vi "collision_fixed_steer2.vi"(6 "safe  dist":dbl=10.0 format="%#_13g", 7 "y":dbl=0.2 format="%#_13g", 8 "obsclose":bool=TRUE, 11 "Max. Vel.":dbl=30.0) -> (0 "collision":bool=TRUE, 1 "collision dist":dbl=nan, 3 "speed limit":dbl)   [LabVIEW 2015]
uses:
  G_ALL.vi
  G_SEN.vi
panel:
  in  "safe time":dbl=0.5
  out "straight":bool
  out "an":dbl=-2.25694
  out "col point":dbl[](array[numeric])=[nan, -21.3]
  out "coldist":dbl=nan
  out "V":dbl=3.694375
  out "Rmax":dbl=-inf
  out "Rmin":dbl=-inf
  out "sensor":dbl[][](array[numeric])=[[-1.5304583967165966, 6.569624655213078, 0.4487461947280802], [-1.5123803553800648, 6.600839252564809, 0.44873888391016814], [-1.5798868335412573, 6.600702497017339, 0.4487279176833], [-1.5216886216577719, 9.603159710523432, 0.44770074776665436], [-1.5313655877780465, 9.6419719017331, 0.4492287086950086], [-1.523389300316294, 12.60341549398873, 0.4466260575335802], [-1.5233893907854144, 12.603416034610877, 0.44887535248893035], [5.990087584334978, 10.963494447794808, 0.45116607548005816], [6.221741073596072, 10.980830526279878, 0.45355671291422156], [5.9936071270446645, 11.240850869489245, 0.45119288181293304], [-1.5383654223459522, 15.592540246828664, 0.4514853145352047], [-9.871601236033586, 12.081252035494268, 0.44840624166361964], [-9.818809426655438, 12.186948767622127, 0.44840258625459123], [-9.44735320706394, 13.283020631001266, 0.4450286438197932], [-9.81432610750644, 13.144511405171443, 0.4483233857256427], [-9.743931372418091, 13.243931372418093, 0.4483209487862904], [-9.847775090309504, 13.52116873622569, 0.44828805010503486], [-9.829415869027697, 13.678658099232255, 0.4482758654082735], [-9.704836591647034, 13.907163096784867, 0.4482661176508645], [-9.822819722231719, 13.851092197505649, 0.4482612437721599], [-9.694719407317505, 14.079929704686844, 0.4482514960147509], [-9.615406741998342, 14.178991062836355, 0.44824905907539864], [-9.607990627804794, 14.359857870824094, 0.4482332189696089], [5.980066449660152, 16.775255255935654, 0.4517740918484479], [-9.552219391192397, 14.488571406471639, 0.4482259081515521], [-9.598842083064628, 14.738800088139001, 0.4481991018186772], [-9.564679561133818, 14.89874122899364, 0.4481869171219159], [-1.4309769895232571, 18.36126424873973, 0.4445424744286406], [-1.50382270432675, 18.434476461172622, 0.4554867688430077], [-9.636584965672458, 15.190112351544258, 0.44815401844066033], [-1.5218566445901764, 18.61357168003814, 0.4518508554380442], [-1.4568554274926686, 18.630022102865794, 0.44814792609227966], [-9.609722299994765, 15.367018743355008, 0.4481393968045468], [-9.56182474777314, 15.520861200018116, 0.4481284305774616], [-9.462716805510386, 15.611725193025839, 0.44812721210778544], [-9.460152536569574, 15.82871081660556, 0.4481064981232912], [-9.472568394095125, 16.0705228348291, 0.44808212872976855], [-9.410096416551857, 16.217015440561624, 0.4480723809723595], [-9.433953229262734, 16.484722663327872, 0.4480443561698085], [-9.366738606084954, 16.63168321360645, 0.44803460841239945], [-9.418125014970215, 16.95047646737776, 0.4479992727917916], [-9.244943886321535, 17.467586586449492, 0.4438771899986423], [-9.42799228252958, 17.477573369517696, 0.4479456601260418], [-9.393967420276597, 17.692736586225667, 0.4479261646112237], [-9.198568680340516, 17.938860587655174, 0.443741939867269], [-9.356898552098706, 17.908360250344202, 0.4479066690964056], [-9.31677513957232, 18.124407561833465, 0.44788717358158747], [-9.358374136887987, 18.476529266946585, 0.44784818255195125], [-9.290024411686542, 18.659942009678325, 0.4478335609158377], [-1.4789544873589022, 21.298658685480213, 0.45652856039547757], [-9.322189086670184, 19.014728027537103, 0.4477945698862015], [-1.4295247135494842, 21.663833685781242, 0.4477799482500879], [-1.5104216938102306, 21.677354630622453, 0.4522224886892644], [-9.308253507600966, 19.302278685191865, 0.4477653266139743], [-9.309999930888686, 19.625392898761945, 0.4477312094630426], [-9.267411332352088, 19.880094075993874, 0.44770684006952], [-9.259863677965905, 20.20523628235378, 0.4476727229185883], [-10.761395333704177, 19.60556627074318, 0.4523601757626673], [-10.65333737048856, 19.74903988749979, 0.45236748658072407], [-9.28550940572247, 20.601780885449482, 0.44762885801024754], [-9.229810855854572, 20.858749546746573, 0.4476044886167249], [-10.560231191577744, 20.2369534672775, 0.45241135148906486], [-10.59794834367646, 20.626093684277787, 0.45245399792772945], [-10.46884427196551, 20.752121422111667, 0.45245887180643396], [-1.481627491326594, 24.688260270230966, 0.4474119704078961], [2.41453226692714, 27.47874111184458, 0.45293651191947765], [2.2051889934181257, 27.49889857639732, 0.45293651191947765], [-1.3984167404305334, 30.183380970562354, 0.44674424902537585], [-9.27247533961122, 28.63414421014917, 0.4597928405932163], [-1.4542170646867847, 33.77509436961648, 0.4536931815883555], [-12.254333639737276, 34.21572986135418, 0.46208843741760597], [9.646867745895442, 40.14137035344789, 0.4546167816028634], [9.346440466929042, 40.30169736837388, 0.4546265293602724], [9.995186075205359, 40.161918033340946, 0.45463018476930084], [9.687603481990763, 40.29609551732546, 0.4639088310777111], [10.355453085480514, 40.217666998138846, 0.4546484618144428], [9.398132099956998, 40.50523366028126, 0.46395635139413954], [9.081977878364448, 40.614980212047534, 0.4546557726324996], [10.748232349142603, 40.37551463322397, 0.45468014202602225], [9.129514514304716, 40.80924640889365, 0.46404042580012833], [-19.28793420922692, 37.246885664560835, 0.4642085746121059], [9.064874855356468, 41.997147100113274, 0.4644571424211163], [-18.15469952147041, 38.74952730488572, 0.4644936965106766], [-17.918417740569364, 39.049489362133144, 0.46455218305397317], [-17.647317560719458, 39.28521999634086, 0.46458508173457747], [-17.399531396582823, 39.572962074832176, 0.464639912868918], [-17.17365632105936, 39.91336172321326, 0.4647166764569947], [-22.342947610202373, 37.578658573998304, 0.4648957914958404], [-22.10962516766409, 37.87326216337433, 0.4649396564033128], [-21.83550453243502, 38.10718015201812, 0.464957933448093], [-21.55372087277477, 38.330424808794795, 0.4649725550839171], [-21.274889895785886, 38.55993347394059, 0.4649908321286973], [-21.029483225367702, 38.84738334349325, 0.46503469703616973], [-20.78067516476939, 39.13321220902357, 0.4650785619436421], [-20.26312153109795, 39.6824069959594, 0.46515898094067487], [-17.797224253682096, 42.105163740090134, 0.46553914347210246], [-17.23352970768187, 42.66617557482583, 0.46564149492287144], [-16.938457745789194, 42.925328193479906, 0.46568535983034387], [17.322133973531134, 42.86754408677865, 0.4657219139199042], [-16.655640004933225, 43.219193196203896, 0.4657438463736404], [-14.15297871173657, 45.19333081613475, 0.4660947656334197], [-14.06731724741144, 46.160481898838114, 0.4664200970305068], [-13.150394836379569, 47.19397827432551, 0.4666796310663852], [-12.785386796883316, 47.364674916290646, 0.46670156352012143], [-12.459115816412385, 47.67669240177406, 0.46677832710819817], [-12.136259424266495, 48.015284147391746, 0.466866056923143], [-9.972349925099477, 49.42985893516836, 0.4671804220933619], [-10.436781004884613, 49.62393525530377, 0.4672864289530869], [-8.077970793908602, 50.511020876260254, 0.46743630072028436], [-10.017137069339602, 51.65924357399377, 0.4679809566547335], [-9.703791968771103, 52.28425658797661, 0.46818200414731537], [-7.575744126121782, 52.72039993287564, 0.4682039366010516], [5.9133064222073175, 53.46127369852273, 0.45613012094061905], [6.356642028184218, 53.46728894444298, 0.4561374317586759], [8.099817339627355, 53.2347435881879, 0.4684196057294576], [8.536907918677832, 53.18187761786749, 0.4684269165473697], [8.977251802514107, 53.14485282772466, 0.4561471795160849], [5.492333795510142, 53.65014189103438, 0.4561471795160849], [9.00928110542982, 53.321977193221436, 0.46850733554440244], [6.832896586246616, 53.7071746478883, 0.4561739858489598], [1.989687447899467, 54.14092718075492, 0.45617520431863595], [-4.637301999436954, 53.96739335484715, 0.45617520431863595], [7.7156976320662, 53.629692461756065, 0.46854023422500674], [10.861374957060782, 53.52445996847586, 0.45623734627211865], [10.444784718162802, 53.715238928850184, 0.4687485925355007], [10.89956629047575, 53.70035858509785, 0.468777835807149], [10.086168974376077, 54.20659560913531, 0.4688984643026981], [15.473538348436962, 53.33293737243348, 0.4690739239325878], [15.075545778895796, 53.5905545371459, 0.46912144424901625], [15.965742273424409, 53.3769646950345, 0.4691433767027524], [16.481810034088696, 53.48266167265918, 0.46923841733560934], [-3.937384054853013, 56.48390194101806, 0.45647372938928826], [14.881305971946919, 54.55544784522514, 0.4694394648281912], [17.54943187485922, 53.75385519804383, 0.4694577418729714], [7.748601530003164, 56.941174491550086, 0.4565797362511117], [20.102739641842973, 53.88791487688127, 0.46983059358648693], [20.59848340778603, 53.84940005470817, 0.46988542472082745], [19.763744907192873, 54.32238571654336, 0.4699329450372559], [21.226563266096697, 54.119607953091055, 0.4700645397596731], [5.15520085107671, 59.60364587126739, 0.47059457405829813], [17.179103122702053, 57.16750291150652, 0.45686607662500267], [5.648602536305274, 59.5963213111867, 0.47060919569412224], [8.262304622246873, 60.484123045962804, 0.47104784476884637], [12.720999304748343, 59.71872759813299, 0.4710697772225826], [7.78089815695139, 60.67295845949319, 0.4710917096763188], [-7.8793393294743455, 61.39629051625974, 0.47135855453010933], [-0.29190538898263213, 70.3993626636003, 0.4581515621333217], [-0.29194900473725677, 70.40935859480476, 0.47445834132482656], [0.8783118563172027, 70.59425088215231, 0.4581759315268444], [0.8790971798389399, 70.65424175329007, 0.4745497265487274], [2.0967743014213513, 72.12797583739979, 0.45836601279632094], [-8.110079882755713, 72.0217189519484, 0.47522232179663776], [5.235520456007894, 83.378606212284, 0.45975384975743505], [-3.240112570543469, 85.96637174877078, 0.4600560302371157], [4.792807940400054, 87.90402618987854, 0.4809028273143153], [4.793942080772132, 87.92399903562121, 0.46030337958137046], [-8.146388565341844, 92.15650677882385, 0.48254410593557473], [-2.802519336461366, 95.22719695016279, 0.4611818962178615], [-3.520704269592428, 164.8515923526585, 0.46966488210309104], [-11.526176157591637, 13.878215627584847, 0.4481101535323196], [-11.789979240029444, 14.885450607304874, 0.44800292820082], [-12.091348233927823, 14.57967932264858, 0.4480017097311439], [-12.030768302326846, 14.71887293974657, 0.4479956173827632], [-11.96142328919889, 14.850966868927898, 0.4479907435040587], [-9.215291856779873, 17.690305061581164, 0.4438150480463897], [-9.236492158493983, 18.281477328454823, 0.44362862218963195], [-9.154174242232312, 18.438254681457707, 0.44359572350902765], [-9.141925218880708, 18.714718570965932, 0.44351164910303886], [-1.414617401462343, 21.474418326335975, 0.4434092976522699], [-9.206745289003786, 19.129951926170946, 0.44336908815375353], [-9.224999383677053, 19.47816763232024, 0.4432557704761165], [-9.183698782366013, 19.732132644809052, 0.44318266229699577], [-9.177445498117294, 20.05654995000434, 0.4430803108462268], [-9.166219172191244, 20.382075606343538, 0.4429779593954578], [-9.070189987043294, 20.558546354351627, 0.44293774989694146], [-9.027184785637978, 20.84106063007659, 0.44285367549095267], [-9.265946030899864, 21.685443023687828, 0.447513103391015], [-9.298762356180521, 22.15043195733767, 0.44746070919494135], [-1.4639438802396605, 27.435270867039012, 0.4412343293234294], [2.307965703554175, 27.469140278750547, 0.44706592501987463], [-9.175563115010997, 28.371452130675763, 0.4532301631114254], [-9.03589297233244, 28.66704646113176, 0.45325818791397643], [-1.4146408027345068, 30.492954521014685, 0.4401194295918389], [-12.23951207009181, 34.17857930362207, 0.45402460534026334], [-12.1194280298934, 38.2047121320138, 0.4544790945294605], [-19.197928435902572, 37.780367863415314, 0.45478736735752184], [-17.90491585155485, 39.02270210519787, 0.4548470723716523], [10.80061477854137, 41.796091299925706, 0.4645448722360611], [-17.64731860873607, 39.285222121508326, 0.4548616940077659], [-17.40387688242602, 39.58197119941406, 0.454881189522584], [-17.173657340946782, 39.91336388568401, 0.4549055589161066], [-22.050119289273855, 37.780749913950906, 0.4549664823999132], [-21.039710335885733, 38.86457357076146, 0.4550140027172824], [-20.498703614653966, 39.36529276030614, 0.4550334982321005], [-19.95622387432352, 39.87539282427752, 0.45505543068627086], [-19.96584246392425, 39.892925198004406, 0.46517360257649903], [-19.71849601752628, 40.19790570184635, 0.46522843371083955], [-17.52126508189382, 42.39576618036936, 0.465593974606443], [-17.2254757973876, 42.64787167133072, 0.4552113948048157], [-16.934511313174397, 42.91614262278823, 0.4552272349106054], [-16.63630544611904, 43.17308550675596, 0.455241856546719], [17.35435473718568, 42.94077134247465, 0.45525038583445193], [-16.368979606633143, 43.51111569166321, 0.4552674444099178], [-16.376551606374004, 43.529624124377364, 0.465809643734849], [-15.482517326111966, 44.36540593305769, 0.46597413713787056], [-14.140121973719118, 45.155456087267005, 0.4553600481053038], [-14.61518532805766, 45.3514634779125, 0.46620442790210076], [-13.967105665492628, 45.85658071417634, 0.4554343747555478], [-12.732220043894518, 47.18226805029135, 0.4555440370263997], [-12.391256444356108, 47.43608121795645, 0.4555623140715417], [-12.081023590373213, 47.8126814545092, 0.45559643122247334], [-11.78806941435407, 48.27422398034609, 0.4669245434664395], [-10.742622242787393, 49.122285505371394, 0.45571096737202976], [-10.786169676183954, 49.30722484276436, 0.46720235454709813], [-10.414711881352668, 49.52640376312698, 0.45574995840166593], [-7.749398570022519, 51.08309165283863, 0.4676227265770421], [-8.230385825965628, 51.39802411465917, 0.45592176262600054], [-10.013064829232125, 51.63966552470979, 0.45599121539754006], [10.051053315658523, 54.03005727127254, 0.45627755577143103], [-9.684327877683424, 54.50882427125252, 0.4563262945584763], [-3.4696359799027956, 56.436415484842804, 0.4564639816318792], [-3.0200247710824435, 56.68432389578455, 0.45649078796475406], [8.73796580135908, 57.15312208792874, 0.45662360115945244], [9.221080416128158, 57.16352701734963, 0.4566345673865376], [11.175859219610716, 57.23001513109769, 0.4566869615826113], [1.9728684167848833, 59.995559676916635, 0.42933597317153727], [-7.872597250938968, 61.34675066002998, 0.4571134259692574], [-8.106554242489338, 71.99193096774223, 0.458403785356281], [3.679295078452094, 87.76971186036354, 0.41916662545584943], [6.462482767471447, 102.0984336178372, 0.48611909589457647], [-4.972546548304975, 22.727410853324365, 0.4427403578133156], [-12.82222968885361, 27.363329920838236, 0.45330083435264107], [-15.118256938908255, 29.423703318743403, 0.4536566274980715], [-18.159279338735963, 38.75841956958901, 0.45483245073553874], [-17.805598505289773, 42.12332889606653, 0.45518215153258856], [-17.541802064902818, 42.441356592102444, 0.45520408398675893], [-15.4754324248608, 44.346705655865925, 0.4553222755453437], [-11.7396957446091, 48.09048791231148, 0.4556183636766437], [-11.088046794705612, 48.813107220413954, 0.4556841610391548], [-9.959619857089923, 49.37122779684034, 0.45571949665976264], [-7.9246084254415505, 52.158920510207636, 0.45600705550332976], [38.47373334497915, 62.182195635275114, 0.47565000464449375], [2.2272997454946832, 105.5757022071159, 0.46244057539330563], [-24.75, -14.799999999999999, 1.31], [-24.75, 28.2, 1.1500000000000001], [-24.5, -14.799999999999999, 1.31], [-24.5, 26.45, 0.36], [-24.5, 26.7, 0.36], [-24.5, 26.95, 0.34], [-24.5, 28.45, 0.29], [-24.5, 28.7, 0.29], [-24.25, -14.799999999999999, 1.32], [-24.0, -14.799999999999999, 1.32], [-24.0, -7.549999999999999, 1.4000000000000001], [-24.0, -1.0499999999999994, 1.44], [-24.0, 6.200000000000001, 1.43], [-23.75, -14.799999999999999, 1.33], [-23.75, -8.049999999999999, 1.4000000000000001], [-23.75, -7.799999999999999, 0.81], [-23.75, -7.549999999999999, 1.41], [-23.75, -1.0499999999999994, 1.44], [-23.75, -0.7999999999999994, 1.44], [-23.75, -0.5499999999999994, 1.44], [-23.75, -0.2999999999999994, 1.44], [-23.75, 5.950000000000001, 0.3], [-23.5, -14.799999999999999, 1.33], [-23.5, -8.049999999999999, 1.41], [-23.5, -7.799999999999999, 1.41], [-23.5, -0.7999999999999994, 1.45], [-23.5, -0.5499999999999994, 1.45], [-23.5, 6.200000000000001, 1.44], [-23.5, 27.7, 0.36], [-23.25, -14.799999999999999, 1.34], [-23.25, 27.7, 1.18], [-23.25, 36.7, 1.02], [-23.0, -14.799999999999999, 1.34], [-23.0, 6.200000000000001, 1.45], [-23.0, 7.450000000000001, 0.34], [-23.0, 27.7, 0.37], [-22.75, -17.55, 1.31], [-22.75, -17.3, 1.31], [-22.75, -17.05, 1.32], [-22.75, -16.8, 1.32], [-22.75, -16.55, 1.32], [-22.75, -16.3, 1.33], [-22.75, -16.05, 1.33], [-22.75, -15.799999999999999, 1.33], [-22.75, -15.549999999999999, 1.34], [-22.75, -15.299999999999999, 1.34], [-22.75, -15.049999999999999, 1.34], [-22.75, -14.799999999999999, 1.35], [-22.75, 6.200000000000001, 1.46], [-22.75, 6.450000000000001, 1.45], [-22.75, 6.700000000000001, 1.45], [-22.75, 6.950000000000001, 1.45], [-22.75, 7.200000000000001, 1.45], [-22.75, 7.450000000000001, 1.45], [-22.75, 7.700000000000001, 1.45], [-22.75, 7.950000000000001, 1.45], [-22.75, 8.200000000000001, 1.44], [-22.75, 8.450000000000001, 1.44], [-22.75, 8.700000000000001, 1.44], [-22.5, 7.700000000000001, 0.37], [-22.5, 7.950000000000001, 0.37], [-20.25, 4.700000000000001, 0.56], [-20.25, 4.950000000000001, 0.56], [-20.0, 8.200000000000001, 1.5], [-20.0, 8.450000000000001, 1.51], [-19.75, 8.450000000000001, 1.51], [-19.0, -9.549999999999999, 0.45], [-18.25, -10.549999999999999, 0.47000000000000003], [-18.25, -10.299999999999999, 0.99], [-18.0, 1.7000000000000006, 0.32], [-18.0, 2.2000000000000006, 0.74], [-18.0, 2.4500000000000006, 0.32], [-17.75, 1.4500000000000006, 0.75], [-17.75, 1.9500000000000006, 0.75], [-17.75, 4.700000000000001, 0.31], [-17.75, 4.950000000000001, 0.31], [-17.5, -5.049999999999999, 0.26], [-17.5, 1.4500000000000006, 0.76], [-17.25, -10.549999999999999, 0.53], [-17.25, -7.049999999999999, 0.65], [-17.25, -6.799999999999999, 0.65], [-17.25, -4.799999999999999, 0.29], [-17.25, -0.2999999999999994, 0.78], [-17.25, -0.04999999999999938, 0.38], [-17.25, 1.4500000000000006, 0.39], [-16.75, -6.299999999999999, 0.28], [-16.75, -5.299999999999999, 0.32], [-16.25, -12.299999999999999, 0.51], [-16.25, -5.799999999999999, 0.76], [-16.25, -0.04999999999999938, 0.48], [-16.25, 4.700000000000001, 0.46], [-16.25, 4.950000000000001, 0.45], [-16.25, 5.200000000000001, 0.45], [-16.0, -5.549999999999999, 0.36], [-16.0, -0.04999999999999938, 0.49], [-16.0, 5.700000000000001, 0.85], [-15.5, -9.799999999999999, 0.22], [-15.5, -9.549999999999999, 0.24], [-15.5, -5.799999999999999, 0.8], [-15.5, -5.299999999999999, 0.42], [-15.5, -5.049999999999999, 0.44], [-15.5, -0.2999999999999994, 0.54], [-15.5, 0.4500000000000006, 0.55], [-15.5, 9.450000000000001, 1.59], [-15.25, -10.049999999999999, 0.66], [-15.25, -9.799999999999999, 0.67], [-15.25, 1.4500000000000006, 0.23], [-15.25, 9.200000000000001, 1.2], [-15.25, 9.950000000000001, 1.59], [-15.0, -21.3, 1.36], [-15.0, 8.950000000000001, 1.61], [-14.75, -19.3, 0.21], [-14.75, -18.8, 0.8300000000000001], [-14.75, -11.799999999999999, 0.62], [-14.75, 4.700000000000001, 0.24], [-14.75, 9.450000000000001, 1.61], [-14.5, -17.8, 0.87], [-14.5, -17.55, 0.33], [-14.5, -17.3, 0.89], [-14.5, -10.299999999999999, 0.68], [-14.5, -10.049999999999999, 0.7000000000000001], [-14.5, -9.799999999999999, 0.71], [-14.5, 8.950000000000001, 0.86], [-14.5, 9.200000000000001, 1.61], [-14.25, -19.05, 0.25], [-14.25, -17.8, 0.33], [-14.25, -17.55, 0.33], [-14.25, -15.049999999999999, 0.46], [-14.25, -6.049999999999999, 0.5], [-14.25, -5.799999999999999, 0.89], [-14.25, -5.299999999999999, 0.53], [-14.25, 0.4500000000000006, 0.34], [-14.25, 8.950000000000001, 1.24], [-14.25, 9.200000000000001, 0.87], [-14.0, -11.049999999999999, 0.26], [-14.0, -10.799999999999999, 0.27], [-14.0, -9.799999999999999, 0.33], [-14.0, -9.549999999999999, 0.35000000000000003], [-14.0, -0.7999999999999994, 0.35000000000000003], [-14.0, -0.2999999999999994, 0.6900000000000001], [-14.0, -0.04999999999999938, 0.36], [-14.0, 0.20000000000000062, 0.6900000000000001], [-14.0, 0.4500000000000006, 0.6900000000000001], [-14.0, 9.200000000000001, 0.87], [-14.0, 9.450000000000001, 1.24], [-13.75, -10.549999999999999, 0.72], [-13.75, -10.299999999999999, 0.31], [-13.75, -10.049999999999999, 0.32], [-13.75, 9.450000000000001, 1.26], [-13.5, -19.05, 0.27], [-13.5, 9.200000000000001, 0.9], [-13.5, 9.450000000000001, 1.26], [-13.5, 19.45, 0.42], [-13.25, -18.8, 0.86], [-13.25, 8.950000000000001, 0.22], [-13.25, 9.200000000000001, 1.28], [-13.25, 9.450000000000001, 1.28], [-13.25, 9.700000000000001, 1.27], [-13.25, 9.950000000000001, 1.27], [-13.25, 14.450000000000001, 1.56], [-13.25, 19.7, 1.47], [-13.25, 27.7, 1.31], [-13.0, -19.8, 0.26], [-13.0, -19.55, 0.27], [-13.0, -19.3, 0.85], [-13.0, 9.450000000000001, 1.28], [-13.0, 9.950000000000001, 1.27], [-13.0, 14.200000000000001, 1.57], [-13.0, 19.7, 1.47], [-12.75, 8.700000000000001, 0.28], [-12.75, 14.450000000000001, 1.58], [-12.75, 19.7, 0.43], [-12.5, 30.7, 1.26], [-12.0, 11.450000000000001, 1.6300000000000001], [-11.75, 10.700000000000001, 1.3], [-11.5, 4.950000000000001, 0.59], [-11.5, 5.200000000000001, 0.58], [-11.5, 5.450000000000001, 0.85], [-11.5, 5.700000000000001, 0.85], [-11.5, 5.950000000000001, 0.27], [-11.5, 10.450000000000001, 0.97], [-11.5, 10.700000000000001, 1.3], [-11.5, 10.950000000000001, 1.31], [-11.5, 11.200000000000001, 1.29], [-11.5, 11.450000000000001, 1.29], [-11.25, 5.200000000000001, 0.32], [-11.25, 6.200000000000001, 0.28], [-11.25, 10.200000000000001, 0.67], [-11.25, 10.450000000000001, 1.32], [-11.25, 10.700000000000001, 1.31], [-11.25, 10.950000000000001, 1.3], [-11.25, 11.200000000000001, 1.3], [-11.0, 3.9500000000000006, 0.68], [-11.0, 10.450000000000001, 0.65], [-11.0, 10.700000000000001, 0.99], [-11.0, 10.950000000000001, 0.98], [-10.75, 3.7000000000000006, 0.45], [-10.75, 3.9500000000000006, 0.7000000000000001], [-10.75, 4.200000000000001, 0.6900000000000001], [-10.75, 4.450000000000001, 0.7000000000000001], [-10.75, 4.700000000000001, 0.6900000000000001], [-10.75, 4.950000000000001, 0.9500000000000001], [-10.75, 5.200000000000001, 0.9500000000000001], [-10.75, 10.700000000000001, 0.67], [-10.75, 10.950000000000001, 1.0], [-10.75, 11.200000000000001, 0.98], [-10.5, 3.9500000000000006, 0.72], [-10.5, 4.200000000000001, 0.48], [-10.5, 4.450000000000001, 0.47000000000000003], [-10.5, 5.200000000000001, 0.7000000000000001], [-10.5, 5.450000000000001, 0.42], [-10.5, 10.450000000000001, 0.72], [-10.5, 10.950000000000001, 0.68], [-10.5, 11.200000000000001, 1.0], [-10.5, 11.450000000000001, 0.99], [-10.5, 11.700000000000001, 0.98], [-10.25, 4.700000000000001, 0.99], [-10.25, 11.200000000000001, 1.01], [-10.25, 11.450000000000001, 0.33], [-10.25, 11.700000000000001, 0.99], [-10.25, 12.200000000000001, 0.96], [-10.25, 15.700000000000001, 0.36], [-10.0, 11.450000000000001, 0.33], [-10.0, 11.700000000000001, 0.99], [-10.0, 11.950000000000001, 1.6600000000000001], [-10.0, 12.200000000000001, 1.6600000000000001], [-10.0, 15.450000000000001, 1.6], [-10.0, 15.700000000000001, 1.59], [-9.75, 11.950000000000001, 1.6600000000000001], [-9.75, 12.200000000000001, 1.6600000000000001], [-9.75, 12.450000000000001, 1.6600000000000001], [-9.75, 12.700000000000001, 0.27], [-9.75, 15.700000000000001, 1.6], [-9.5, 11.950000000000001, 0.66], [-9.5, 12.200000000000001, 0.67], [-9.5, 12.700000000000001, 0.27], [-9.5, 15.950000000000001, 0.38], [-9.5, 16.2, 0.36], [-8.5, -10.549999999999999, 1.31], [-8.5, -1.0499999999999994, 1.79], [-8.5, -0.5499999999999994, 1.79], [-8.5, 6.450000000000001, 0.38], [-8.25, -14.049999999999999, 1.59], [-8.25, -10.549999999999999, 1.32], [-8.25, -1.5499999999999994, 1.59], [-8.25, -1.2999999999999994, 1.59], [-8.25, -1.0499999999999994, 1.8], [-8.25, -0.7999999999999994, 1.8], [-8.25, 2.4500000000000006, 1.8], [-8.25, 6.700000000000001, 1.31], [-8.0, -14.049999999999999, 1.59], [-8.0, -13.799999999999999, 1.6], [-8.0, -10.549999999999999, 1.6600000000000001], [-8.0, -10.299999999999999, 1.6600000000000001], [-8.0, -3.0499999999999994, 1.57], [-8.0, -2.7999999999999994, 1.79], [-8.0, -1.2999999999999994, 1.8], [-8.0, -1.0499999999999994, 1.6], [-8.0, -0.7999999999999994, 1.8], [-8.0, 2.4500000000000006, 1.81], [-8.0, 2.7000000000000006, 1.81], [-8.0, 2.9500000000000006, 1.81], [-8.0, 6.700000000000001, 1.78], [-8.0, 8.950000000000001, 0.46], [-8.0, 9.200000000000001, 0.43], [-8.0, 30.2, 1.3], [-7.75, -14.049999999999999, 0.38], [-7.75, -10.799999999999999, 0.32], [-7.75, -10.549999999999999, 0.66], [-7.75, -3.0499999999999994, 1.79], [-7.75, -2.7999999999999994, 1.79], [-7.75, -1.5499999999999994, 0.24], [-7.75, -1.2999999999999994, 1.8], [-7.75, -1.0499999999999994, 0.25], [-7.75, 2.7000000000000006, 1.81], [-7.75, 6.700000000000001, 1.78], [-7.75, 6.950000000000001, 0.21], [-7.75, 9.200000000000001, 0.2], [-7.5, -16.05, 1.55], [-7.5, -10.799999999999999, 1.6600000000000001], [-7.5, -10.549999999999999, 1.67], [-7.5, -2.5499999999999994, 0.2], [-7.5, 2.7000000000000006, 0.21], [-7.5, 2.9500000000000006, 0.21], [-7.5, 6.700000000000001, 1.78], [-7.5, 6.950000000000001, 1.78], [-7.5, 7.200000000000001, 1.78], [-7.5, 7.450000000000001, 0.42], [-6.75, -13.549999999999999, 0.85], [-6.75, -13.299999999999999, 1.62], [-6.5, -13.549999999999999, 0.48], [-6.5, -13.299999999999999, 1.62], [-6.25, -13.299999999999999, 1.25], [-5.25, -7.799999999999999, 0.24], [-5.25, -4.049999999999999, 0.22], [-5.25, -3.7999999999999994, 0.22], [-5.25, -3.0499999999999994, 0.2], [-5.25, -2.7999999999999994, 0.21], [-5.0, -8.299999999999999, 0.21], [-5.0, -5.299999999999999, 0.22], [-5.0, -3.0499999999999994, 0.23], [-4.75, -8.549999999999999, 0.43], [-4.75, -5.549999999999999, 0.39], [-4.75, -2.7999999999999994, 0.5], [-4.75, -2.5499999999999994, 0.51], [-4.75, 0.20000000000000062, 0.46], [-4.75, 0.4500000000000006, 0.46], [-1.75, 6.700000000000001, 0.45], [-1.5, 6.700000000000001, 0.44], [-1.5, 9.700000000000001, 0.42], [-1.5, 12.700000000000001, 0.41000000000000003], [1.25, -16.3, 0.75], [1.5, -16.8, 0.28], [1.75, 3.7000000000000006, 0.3], [1.75, 3.9500000000000006, 0.28], [1.75, 4.200000000000001, 0.28], [1.75, 4.450000000000001, 0.27], [1.75, 4.950000000000001, 0.26], [1.75, 5.200000000000001, 0.24], [1.75, 5.450000000000001, 0.27], [1.75, 5.700000000000001, 0.28], [1.75, 5.950000000000001, 0.26], [1.75, 6.200000000000001, 0.26], [1.75, 6.700000000000001, 0.27], [1.75, 7.200000000000001, 0.27], [1.75, 7.450000000000001, 0.22], [1.75, 7.950000000000001, 0.25], [1.75, 8.450000000000001, 0.27], [1.75, 8.700000000000001, 0.24], [1.75, 9.450000000000001, 0.26], [2.0, 3.7000000000000006, 0.29], [2.0, 3.9500000000000006, 0.29], [2.0, 4.200000000000001, 0.28], [2.0, 4.450000000000001, 0.28], [2.0, 4.700000000000001, 0.28], [2.0, 4.950000000000001, 0.27], [2.0, 5.200000000000001, 0.27], [2.0, 5.450000000000001, 0.28], [2.0, 5.700000000000001, 0.29], [2.0, 6.200000000000001, 0.27], [2.0, 6.450000000000001, 0.28], [2.0, 6.700000000000001, 0.28], [2.0, 7.200000000000001, 0.27], [2.0, 7.700000000000001, 0.27], [2.0, 8.450000000000001, 0.28], [2.0, 9.200000000000001, 0.27], [2.0, 9.450000000000001, 0.26], [2.0, 10.450000000000001, 0.26], [2.0, 11.700000000000001, 0.26], [2.25, -14.549999999999999, 0.87], [2.25, -14.299999999999999, 0.51], [2.25, 4.450000000000001, 0.29], [2.25, 4.700000000000001, 0.28], [2.25, 4.950000000000001, 0.28], [2.25, 5.200000000000001, 0.29], [2.25, 5.450000000000001, 0.29], [2.25, 5.700000000000001, 0.28], [2.5, -14.549999999999999, 0.87], [2.5, -14.299999999999999, 0.88], [2.5, -14.049999999999999, 0.89], [2.75, -13.799999999999999, 0.54], [3.0, -13.549999999999999, 0.92], [3.0, -2.5499999999999994, 0.2], [3.25, -13.799999999999999, 0.91], [3.25, -13.549999999999999, 0.56], [3.25, -2.2999999999999994, 0.58], [3.25, -2.0499999999999994, 0.45], [3.5, -13.799999999999999, 0.91], [3.5, -2.0499999999999994, 0.5700000000000001], [3.5, -1.7999999999999994, 0.22], [3.75, -14.049999999999999, 0.89], [3.75, -13.799999999999999, 0.9], [3.75, -2.2999999999999994, 0.22], [3.75, -2.0499999999999994, 0.22], [3.75, -1.7999999999999994, 0.22], [4.0, -14.049999999999999, 0.88], [4.0, -4.049999999999999, 0.22], [4.0, -3.5499999999999994, 0.2], [4.25, -3.7999999999999994, 0.56], [4.5, -4.549999999999999, 0.24], [4.5, -4.299999999999999, 0.25], [4.5, -3.7999999999999994, 0.22], [4.5, -3.5499999999999994, 0.24], [4.75, -4.299999999999999, 1.48], [4.75, -4.049999999999999, 1.82], [5.0, -4.049999999999999, 1.83], [5.0, -3.7999999999999994, 1.83], [5.0, -3.5499999999999994, 0.3], [5.25, -4.799999999999999, 0.28], [5.25, -4.549999999999999, 0.52], [5.25, -4.299999999999999, 0.74], [5.25, -4.049999999999999, 1.82], [5.25, -3.7999999999999994, 1.48], [5.25, -3.5499999999999994, 0.31], [5.25, 1.7000000000000006, 0.36], [5.25, 1.9500000000000006, 0.36], [5.25, 2.2000000000000006, 0.36], [5.25, 2.4500000000000006, 0.36], [5.25, 3.7000000000000006, 0.37], [5.25, 3.9500000000000006, 0.36], [5.25, 4.450000000000001, 0.38], [5.25, 4.700000000000001, 0.38], [5.25, 5.700000000000001, 0.39], [5.25, 5.950000000000001, 0.37], [5.25, 8.450000000000001, 0.36], [5.5, -7.049999999999999, 0.35000000000000003], [5.5, -6.799999999999999, 0.38], [5.5, -6.549999999999999, 0.39], [5.5, -5.549999999999999, 0.34], [5.5, -5.299999999999999, 0.36], [5.5, -5.049999999999999, 0.37], [5.5, -4.299999999999999, 0.33], [5.5, -4.049999999999999, 0.35000000000000003], [5.5, -3.7999999999999994, 0.37], [5.5, -3.0499999999999994, 0.34], [5.5, -2.7999999999999994, 0.36], [5.5, -2.5499999999999994, 0.38], [5.5, -1.7999999999999994, 0.35000000000000003], [5.5, -1.5499999999999994, 0.36], [5.5, -1.2999999999999994, 0.36], [5.5, -0.7999999999999994, 0.33], [5.5, -0.5499999999999994, 0.33], [5.5, -0.2999999999999994, 0.45], [5.5, -0.04999999999999938, 0.34], [5.5, 0.20000000000000062, 0.34], [5.5, 1.7000000000000006, 0.38], [5.5, 1.9500000000000006, 0.52], [5.5, 2.2000000000000006, 0.51], [5.5, 2.4500000000000006, 0.5], [5.5, 2.7000000000000006, 0.49], [5.5, 2.9500000000000006, 0.47000000000000003], [5.5, 3.2000000000000006, 0.46], [5.5, 3.4500000000000006, 0.45], [5.5, 3.7000000000000006, 0.42], [5.5, 3.9500000000000006, 0.54], [5.5, 4.200000000000001, 0.53], [5.5, 4.450000000000001, 0.5], [5.5, 4.700000000000001, 0.47000000000000003], [5.5, 4.950000000000001, 0.44], [5.5, 5.200000000000001, 0.41000000000000003], [5.5, 5.450000000000001, 0.52], [5.5, 5.700000000000001, 0.51], [5.5, 6.200000000000001, 0.45], [5.5, 6.450000000000001, 0.41000000000000003], [5.5, 6.700000000000001, 0.39], [5.5, 7.700000000000001, 0.41000000000000003], [5.5, 7.950000000000001, 0.4], [5.5, 8.200000000000001, 0.38], [5.5, 8.700000000000001, 0.5], [5.5, 9.700000000000001, 0.38], [5.75, -7.049999999999999, 0.5700000000000001], [5.75, -6.799999999999999, 0.59], [5.75, -6.549999999999999, 0.61], [5.75, -6.299999999999999, 0.62], [5.75, -6.049999999999999, 0.47000000000000003], [5.75, -5.799999999999999, 0.5], [5.75, -5.549999999999999, 0.53], [5.75, -5.299999999999999, 0.56], [5.75, -5.049999999999999, 0.58], [5.75, -4.799999999999999, 0.6], [5.75, -4.549999999999999, 0.45], [5.75, -4.299999999999999, 0.49], [5.75, -4.049999999999999, 0.52], [5.75, -3.7999999999999994, 0.55], [5.75, -3.5499999999999994, 0.5700000000000001], [5.75, -3.2999999999999994, 0.59], [5.75, -3.0499999999999994, 0.47000000000000003], [5.75, -2.7999999999999994, 0.51], [5.75, -2.5499999999999994, 0.54], [5.75, -2.2999999999999994, 0.56], [5.75, -2.0499999999999994, 0.58], [5.75, -1.7999999999999994, 0.6], [5.75, -1.5499999999999994, 0.59], [5.75, -1.2999999999999994, 0.52], [5.75, -1.0499999999999994, 0.54], [5.75, -0.7999999999999994, 0.55], [5.75, -0.5499999999999994, 0.5700000000000001], [5.75, -0.2999999999999994, 0.5700000000000001], [5.75, -0.04999999999999938, 0.5700000000000001], [5.75, 0.20000000000000062, 0.58], [5.75, 0.4500000000000006, 0.58], [5.75, 0.7000000000000006, 0.51], [5.75, 0.9500000000000006, 0.52], [5.75, 1.2000000000000006, 0.52], [5.75, 1.4500000000000006, 0.52], [5.75, 1.7000000000000006, 0.52], [5.75, 1.9500000000000006, 0.52], [5.75, 2.2000000000000006, 0.51], [5.75, 2.4500000000000006, 0.58], [5.75, 2.7000000000000006, 0.58], [5.75, 2.9500000000000006, 0.58], [5.75, 3.2000000000000006, 0.58], [5.75, 3.4500000000000006, 0.5700000000000001], [5.75, 3.7000000000000006, 0.56], [5.75, 3.9500000000000006, 0.54], [5.75, 4.700000000000001, 0.58], [5.75, 4.950000000000001, 0.56], [5.75, 5.200000000000001, 0.55], [5.75, 5.450000000000001, 0.53], [5.75, 6.450000000000001, 0.56], [5.75, 6.700000000000001, 0.54], [5.75, 6.950000000000001, 0.51], [5.75, 7.450000000000001, 0.46], [5.75, 7.700000000000001, 0.42], [5.75, 7.950000000000001, 0.55], [5.75, 8.200000000000001, 0.54], [5.75, 8.450000000000001, 0.52], [5.75, 9.950000000000001, 0.54], [5.75, 10.700000000000001, 0.48], [5.75, 10.950000000000001, 0.45], [5.75, 11.200000000000001, 0.42], [5.75, 11.450000000000001, 0.39], [6.0, -6.299999999999999, 0.63], [6.0, -6.049999999999999, 0.65], [6.0, -5.799999999999999, 0.66], [6.0, -4.549999999999999, 0.6], [6.0, -4.299999999999999, 0.6], [6.0, -3.2999999999999994, 0.59], [6.0, -3.0499999999999994, 0.59], [6.0, -2.7999999999999994, 0.6], [6.0, -2.5499999999999994, 0.62], [6.0, -1.5499999999999994, 0.59], [6.0, -1.2999999999999994, 0.61], [6.0, -1.0499999999999994, 0.59], [6.0, 0.20000000000000062, 0.58], [6.0, 0.4500000000000006, 0.58], [6.0, 0.7000000000000006, 0.59], [6.0, 0.9500000000000006, 0.59], [6.0, 1.2000000000000006, 0.59], [6.0, 1.4500000000000006, 0.59], [6.0, 1.7000000000000006, 0.59], [6.0, 1.9500000000000006, 0.59], [6.0, 3.7000000000000006, 0.62], [6.0, 3.9500000000000006, 0.61], [6.0, 7.450000000000001, 0.58], [6.0, 7.700000000000001, 0.58], [6.0, 7.950000000000001, 0.56], [6.0, 9.700000000000001, 0.55], [6.0, 10.950000000000001, 0.68], [6.0, 11.200000000000001, 0.66], [6.0, 11.450000000000001, 0.64], [6.0, 11.700000000000001, 0.61], [6.25, -14.799999999999999, 0.78], [6.25, -14.549999999999999, 1.6], [6.25, -6.299999999999999, 1.53], [6.25, -5.799999999999999, 0.67], [6.25, -5.549999999999999, 0.67], [6.25, -4.299999999999999, 0.61], [6.25, -4.049999999999999, 0.63], [6.25, -3.7999999999999994, 0.66], [6.25, -0.2999999999999994, 0.62], [6.25, -0.04999999999999938, 0.64], [6.25, 0.20000000000000062, 0.66], [6.25, 0.4500000000000006, 0.67], [6.25, 0.7000000000000006, 0.67], [6.25, 0.9500000000000006, 0.67], [6.25, 1.2000000000000006, 0.65], [6.25, 1.4500000000000006, 0.65], [6.25, 3.7000000000000006, 0.61], [6.25, 4.950000000000001, 0.61], [6.25, 5.200000000000001, 0.62], [6.25, 5.450000000000001, 0.61], [6.25, 5.700000000000001, 0.59], [6.25, 6.700000000000001, 0.63], [6.25, 6.950000000000001, 0.62], [6.25, 7.200000000000001, 0.61], [6.25, 7.450000000000001, 0.59], [6.25, 8.950000000000001, 0.61], [6.25, 9.200000000000001, 0.6], [6.25, 10.700000000000001, 0.7000000000000001], [6.25, 10.950000000000001, 0.68], [6.5, -14.549999999999999, 0.79], [6.5, -6.299999999999999, 1.53], [6.5, -5.299999999999999, 1.78], [6.5, -5.049999999999999, 1.78], [6.5, -4.799999999999999, 0.72], [6.5, -4.049999999999999, 0.8], [6.5, -3.7999999999999994, 0.64], [6.5, -3.5499999999999994, 0.66], [6.5, -0.04999999999999938, 0.75], [6.5, 0.20000000000000062, 0.77], [6.5, 0.4500000000000006, 0.77], [6.5, 0.7000000000000006, 0.77], [6.5, 0.9500000000000006, 0.77], [6.5, 1.4500000000000006, 0.64], [6.5, 1.7000000000000006, 0.64], [6.5, 1.9500000000000006, 0.64], [6.5, 2.2000000000000006, 0.63], [6.5, 2.4500000000000006, 0.62], [6.5, 2.7000000000000006, 0.62], [6.5, 3.7000000000000006, 0.68], [6.5, 3.9500000000000006, 1.83], [6.5, 4.200000000000001, 1.67], [6.5, 4.450000000000001, 1.6600000000000001], [6.5, 4.700000000000001, 1.6600000000000001], [6.5, 4.950000000000001, 1.6500000000000001], [6.5, 5.200000000000001, 1.6500000000000001], [6.5, 5.450000000000001, 1.6400000000000001], [6.5, 5.700000000000001, 1.6300000000000001], [6.5, 5.950000000000001, 1.6300000000000001], [6.5, 6.200000000000001, 1.62], [6.5, 6.450000000000001, 0.84], [6.5, 6.700000000000001, 0.8200000000000001], [6.5, 6.950000000000001, 1.8], [6.5, 7.200000000000001, 1.79], [6.5, 7.450000000000001, 1.79], [6.5, 7.700000000000001, 1.79], [6.5, 7.950000000000001, 1.78], [6.5, 8.200000000000001, 1.78], [6.5, 8.450000000000001, 1.77], [6.5, 8.700000000000001, 1.77], [6.5, 8.950000000000001, 1.77], [6.5, 11.200000000000001, 1.72], [6.5, 11.450000000000001, 0.88], [6.5, 16.7, 1.61], [6.75, -19.8, 1.48], [6.75, -14.299999999999999, 0.8], [6.75, -14.049999999999999, 1.6], [6.75, -6.549999999999999, 1.75], [6.75, -5.299999999999999, 1.77], [6.75, -5.049999999999999, 1.78], [6.75, -4.799999999999999, 0.72], [6.75, -4.049999999999999, 0.79], [6.75, -3.7999999999999994, 0.81], [6.75, -3.5499999999999994, 0.81], [6.75, -3.2999999999999994, 0.81], [6.75, -3.0499999999999994, 0.67], [6.75, -0.2999999999999994, 0.6900000000000001], [6.75, -0.04999999999999938, 0.71], [6.75, 0.20000000000000062, 0.85], [6.75, 0.4500000000000006, 1.84], [6.75, 0.7000000000000006, 1.52], [6.75, 1.2000000000000006, 0.74], [6.75, 1.4500000000000006, 0.71], [6.75, 1.7000000000000006, 1.84], [6.75, 2.2000000000000006, 1.84], [6.75, 2.4500000000000006, 1.84], [6.75, 2.7000000000000006, 1.84], [6.75, 2.9500000000000006, 1.84], [6.75, 3.2000000000000006, 1.84], [6.75, 3.4500000000000006, 1.83], [6.75, 3.7000000000000006, 1.83], [6.75, 3.9500000000000006, 1.83], [6.75, 4.200000000000001, 1.83], [6.75, 4.450000000000001, 1.83], [6.75, 4.700000000000001, 1.82], [6.75, 4.950000000000001, 1.82], [6.75, 5.200000000000001, 1.82], [6.75, 5.450000000000001, 1.82], [6.75, 5.700000000000001, 1.81], [6.75, 5.950000000000001, 1.81], [6.75, 6.200000000000001, 1.81], [6.75, 6.450000000000001, 1.8], [6.75, 6.700000000000001, 1.8], [6.75, 6.950000000000001, 1.79], [6.75, 7.200000000000001, 1.59], [6.75, 7.450000000000001, 1.58], [6.75, 7.700000000000001, 1.57], [6.75, 7.950000000000001, 1.57], [6.75, 8.200000000000001, 0.9], [6.75, 8.450000000000001, 1.54], [6.75, 8.700000000000001, 1.53], [6.75, 11.200000000000001, 1.72], [6.75, 16.7, 0.8300000000000001], [7.0, -14.299999999999999, 0.79], [7.0, -7.049999999999999, 0.97], [7.0, -6.799999999999999, 1.75], [7.0, -6.549999999999999, 0.75], [7.0, -5.799999999999999, 1.76], [7.0, -5.549999999999999, 1.77], [7.0, -5.299999999999999, 1.77], [7.0, -3.2999999999999994, 0.81], [7.0, -0.04999999999999938, 0.8200000000000001], [7.0, 0.20000000000000062, 0.85], [7.0, 0.4500000000000006, 1.83], [7.0, 0.7000000000000006, 0.86], [7.0, 0.9500000000000006, 0.85], [7.0, 1.4500000000000006, 0.7000000000000001], [7.0, 1.7000000000000006, 0.6900000000000001], [7.0, 1.9500000000000006, 0.6900000000000001], [7.0, 2.2000000000000006, 0.68], [7.0, 2.4500000000000006, 0.67], [7.0, 2.7000000000000006, 0.81], [7.0, 2.9500000000000006, 1.67], [7.0, 3.2000000000000006, 1.6600000000000001], [7.0, 3.4500000000000006, 1.6600000000000001], [7.0, 3.7000000000000006, 1.6500000000000001], [7.0, 3.9500000000000006, 1.6500000000000001], [7.0, 8.450000000000001, 1.31], [7.0, 11.450000000000001, 0.87], [7.25, -5.299999999999999, 1.77], [7.25, -3.5499999999999994, 0.96], [7.25, -3.2999999999999994, 0.79], [7.25, 2.7000000000000006, 0.9500000000000001], [7.25, 2.9500000000000006, 1.6600000000000001], [7.25, 3.2000000000000006, 1.48], [7.25, 3.4500000000000006, 1.6500000000000001], [7.25, 3.7000000000000006, 1.6400000000000001], [7.25, 3.9500000000000006, 1.6400000000000001], [7.25, 4.200000000000001, 1.27], [7.5, -5.299999999999999, 1.76], [7.5, -3.5499999999999994, 0.9500000000000001], [7.5, 2.7000000000000006, 0.93], [7.5, 2.9500000000000006, 1.1], [7.5, 3.4500000000000006, 1.27], [7.5, 3.9500000000000006, 1.6300000000000001], [7.5, 4.200000000000001, 1.26], [7.75, -5.299999999999999, 1.76], [7.75, 2.4500000000000006, 0.71], [7.75, 2.7000000000000006, 0.87], [7.75, 2.9500000000000006, 1.62], [7.75, 3.2000000000000006, 1.45], [7.75, 4.200000000000001, 1.23], [8.0, -5.299999999999999, 1.75], [8.0, -5.049999999999999, 0.79], [8.0, 2.7000000000000006, 1.43], [8.0, 2.9500000000000006, 1.62], [8.0, 3.9500000000000006, 1.02], [8.0, 4.200000000000001, 1.41], [8.25, -5.299999999999999, 1.75], [8.25, -5.049999999999999, 1.75], [8.25, -4.799999999999999, 0.79], [8.25, 2.4500000000000006, 1.6], [8.25, 2.7000000000000006, 1.61], [8.25, 2.9500000000000006, 1.61], [8.5, -5.299999999999999, 1.75], [8.5, -5.049999999999999, 1.75], [8.5, 2.7000000000000006, 1.6], [8.5, 2.9500000000000006, 1.6], [8.5, 3.2000000000000006, 1.3900000000000001], [8.75, -5.049999999999999, 1.74], [8.75, 2.9500000000000006, 0.97], [8.75, 3.2000000000000006, 1.3800000000000001], [9.0, -5.299999999999999, 1.48], [9.0, -5.049999999999999, 1.74], [9.25, -5.049999999999999, 1.73], [9.25, 2.7000000000000006, 0.7000000000000001], [9.25, 2.9500000000000006, 0.91], [9.5, -5.299999999999999, 1.73], [9.5, -5.049999999999999, 1.73], [9.75, -5.299999999999999, 1.45], [9.75, -5.049999999999999, 1.72], [10.0, -5.299999999999999, 1.72], [10.0, -5.049999999999999, 1.16], [10.0, -4.799999999999999, 0.9], [10.25, -15.299999999999999, 1.54], [10.25, -5.299999999999999, 1.71], [10.25, -5.049999999999999, 1.71], [10.25, 15.700000000000001, 1.17], [10.5, -15.299999999999999, 1.08], [10.5, -15.049999999999999, 1.54], [10.5, -14.799999999999999, 1.55], [10.5, -14.549999999999999, 1.55], [10.5, -14.299999999999999, 1.56], [10.5, -14.049999999999999, 1.56], [10.5, -13.799999999999999, 1.57], [10.5, -13.549999999999999, 1.57], [10.5, -5.049999999999999, 1.42], [10.5, 2.9500000000000006, 1.0], [10.5, 3.2000000000000006, 1.01], [10.5, 15.450000000000001, 0.77], [10.5, 15.700000000000001, 0.76], [10.5, 18.95, 0.5700000000000001], [10.75, -13.549999999999999, 1.57], [10.75, -5.299999999999999, 1.7], [10.75, -5.049999999999999, 1.7], [10.75, 2.9500000000000006, 0.99], [10.75, 3.2000000000000006, 0.99], [10.75, 14.950000000000001, 0.79], [10.75, 15.200000000000001, 0.78], [10.75, 18.7, 0.58], [10.75, 19.2, 1.03], [11.0, -13.549999999999999, 1.56], [11.0, -5.299999999999999, 1.4000000000000001], [11.0, -5.049999999999999, 1.4000000000000001], [11.0, 14.700000000000001, 1.6], [11.0, 14.950000000000001, 1.59], [11.0, 16.95, 1.11], [11.25, -13.549999999999999, 1.56], [11.25, 14.700000000000001, 0.78], [11.25, 14.950000000000001, 0.78], [11.25, 19.2, 1.01], [11.25, 19.7, 1.5], [11.5, -13.549999999999999, 1.56], [11.5, -3.0499999999999994, 0.84], [11.5, -2.7999999999999994, 1.71], [11.5, -2.5499999999999994, 1.71], [11.5, -2.2999999999999994, 1.72], [11.5, -2.0499999999999994, 1.72], [11.5, -1.7999999999999994, 1.72], [11.5, -1.5499999999999994, 1.72], [11.5, 13.950000000000001, 1.2], [11.5, 14.200000000000001, 1.2], [11.5, 14.450000000000001, 1.19], [11.5, 14.700000000000001, 1.18], [11.5, 18.95, 1.02], [11.5, 19.2, 1.5], [11.75, -13.549999999999999, 1.56], [11.75, -5.549999999999999, 1.36], [11.75, -2.7999999999999994, 1.71], [11.75, -1.7999999999999994, 1.43], [11.75, -1.5499999999999994, 1.72], [11.75, -1.2999999999999994, 0.87], [11.75, 13.700000000000001, 1.2], [11.75, 13.950000000000001, 1.2], [11.75, 15.950000000000001, 1.1300000000000001], [11.75, 16.2, 1.56], [12.0, -13.549999999999999, 1.55], [12.0, -5.549999999999999, 1.35], [12.0, -1.5499999999999994, 1.71], [12.0, 13.700000000000001, 1.2], [12.0, 18.7, 1.02], [12.25, -5.549999999999999, 1.34], [12.25, -5.299999999999999, 1.01], [12.25, -1.5499999999999994, 1.7], [12.5, -5.549999999999999, 1.33], [12.5, -5.299999999999999, 1.01], [12.75, -5.299999999999999, 0.99], [12.75, 17.2, 1.52], [13.0, 16.7, 1.53], [13.0, 16.95, 1.53], [14.25, -4.299999999999999, 0.93], [14.25, -4.049999999999999, 0.93], [14.25, -3.7999999999999994, 0.93], [14.5, -4.549999999999999, 1.26], [14.5, -4.299999999999999, 1.27], [14.5, -4.049999999999999, 1.27], [14.5, -3.7999999999999994, 1.27], [14.5, -2.0499999999999994, 1.3], [14.5, -1.7999999999999994, 1.3], [14.5, -1.5499999999999994, 1.3], [14.5, -1.2999999999999994, 1.31], [14.5, -1.0499999999999994, 1.31], [14.5, -0.7999999999999994, 1.31], [14.5, -0.2999999999999994, 1.31], [14.5, -0.04999999999999938, 1.32], [14.5, 0.20000000000000062, 1.32], [14.5, 0.4500000000000006, 1.32], [14.5, 0.7000000000000006, 1.32], [14.5, 0.9500000000000006, 1.32], [14.5, 1.2000000000000006, 1.32], [14.5, 1.4500000000000006, 1.32], [14.5, 1.7000000000000006, 1.32], [14.5, 1.9500000000000006, 1.32], [14.5, 2.2000000000000006, 1.32], [14.5, 2.4500000000000006, 1.32], [14.5, 2.7000000000000006, 1.32], [14.5, 2.9500000000000006, 1.32], [14.5, 3.2000000000000006, 1.32], [14.5, 3.4500000000000006, 0.98], [14.5, 3.7000000000000006, 0.98], [16.0, -7.049999999999999, 1.1500000000000001], [16.25, -7.049999999999999, 1.57], [16.25, -6.799999999999999, 1.57], [16.25, -6.549999999999999, 1.1500000000000001], [16.5, -6.799999999999999, 1.57]]
  out "R":dbl=-inf
  out "margin":dbl=0.3
  out "aw":dbl=0.9025
  out "af":dbl=3.5
  out "ar":dbl=0.75
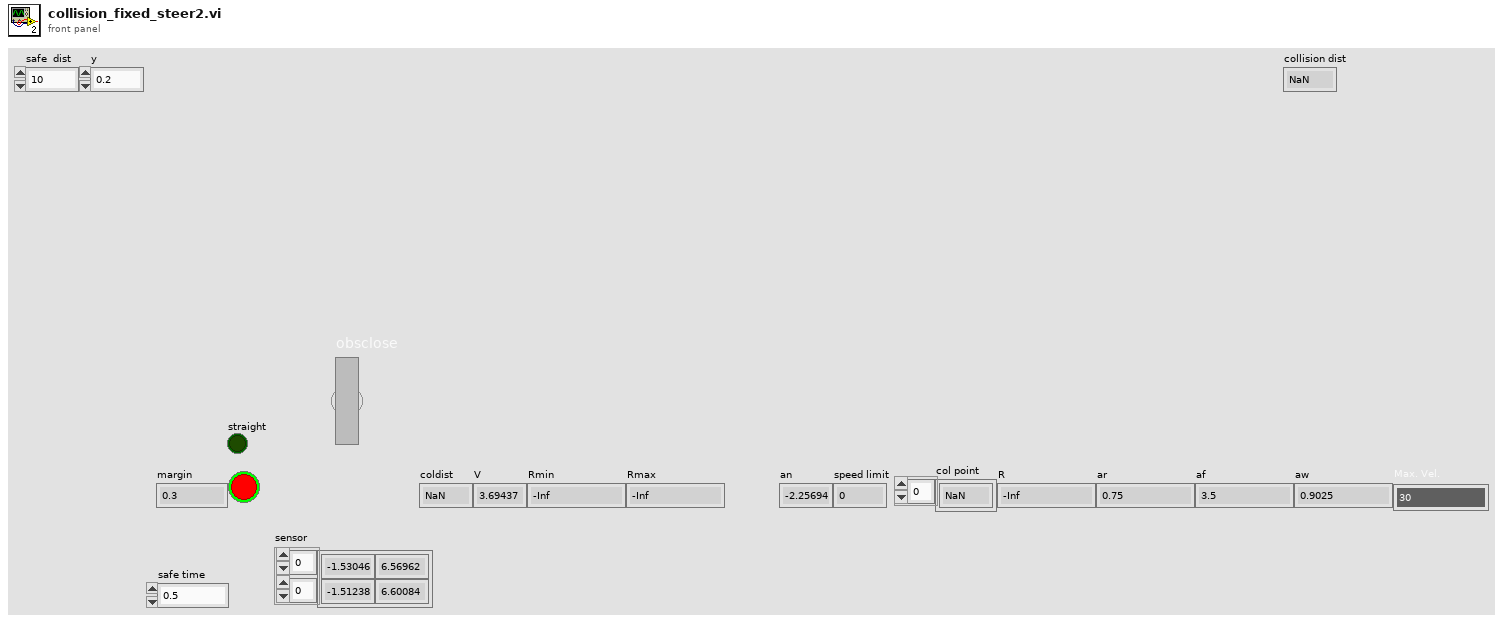
[diagram p1: front panel]
types:
  T1 = cluster{"C_Wheel base":dbl, "ratio_steer":dbl, "Overall width":dbl, "af":dbl, "turn radius":dbl, "eval":dbl, "ap":dbl, "an":dbl, "Vmax":dbl, "mu":dbl, "Vlast":dbl}
  T2 = cluster{"Steer_input":dbl, "Steer_output":dbl, "VS_des":dbl, "VS_can":dbl, "heading":dbl, "auto":bool, "run":bool, "x":dbl, "y":dbl, "slam_y":dbl, "slam_x":dbl, "slam_heading":dbl}
  T3 = cluster{i16, "Real Matrix Element":dbl, "Real Matrix Element":dbl}[]
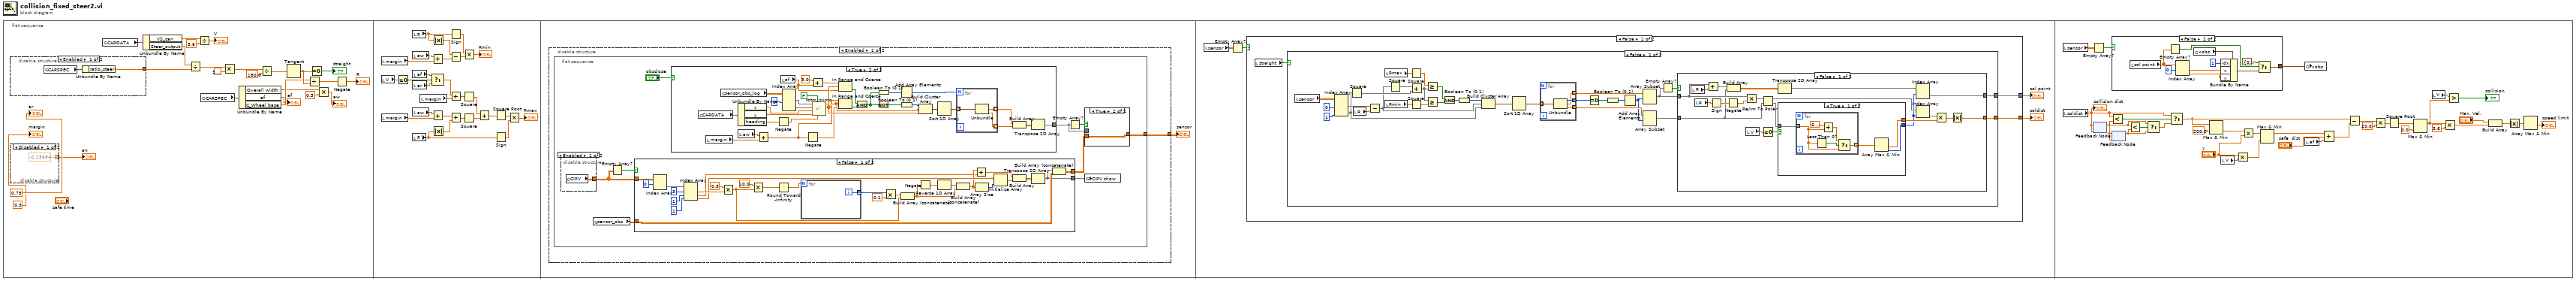
[diagram p0: block diagram]
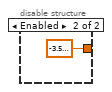
[diagram p2: hidden frame]
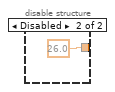
[diagram p3: hidden frame]
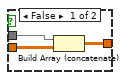
[diagram p7: hidden frame]
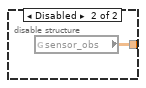
[diagram p8: hidden frame]
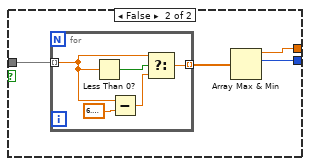
[diagram p9: hidden frame]
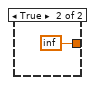
[diagram p10: hidden frame]
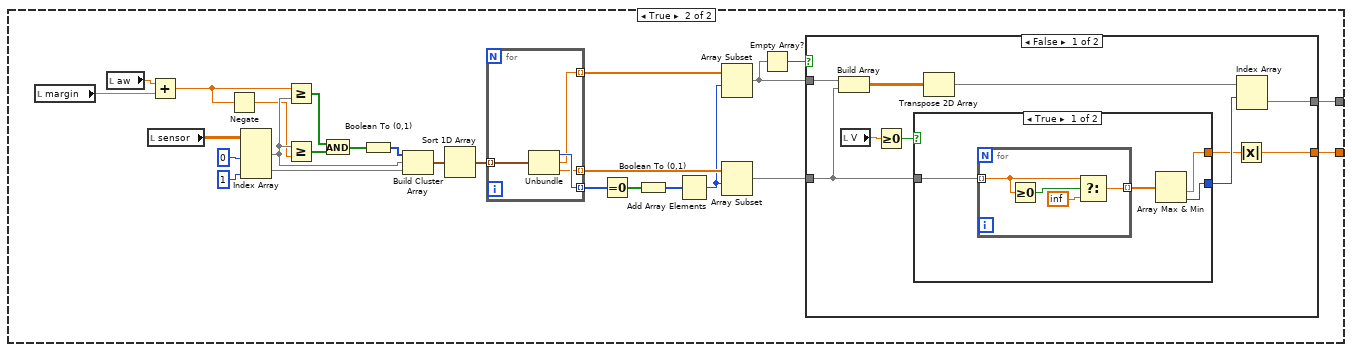
[diagram p11: hidden frame]
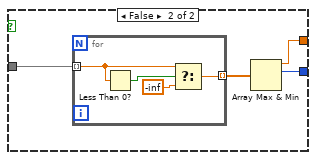
[diagram p12: hidden frame]
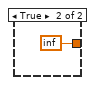
[diagram p13: hidden frame]
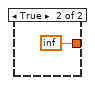
[diagram p14: hidden frame]
diagram:
  n1 = flat-sequence {
    frame #0 {
      n2 = disable-structure shown="Enabled" {
        disable-tunnel: [w27 26.0 ("ratio_steer")] -> w20
        frame Enabled {
          n3 = global read "G_ALL.vi" "CARSPEC"() -> (w28:T1)
          n4 = Unbundle By Name(w28) -> ("ratio_steer"=w27:dbl)
        }
        frame Disabled {
        }
      }
      n5 = disable-structure shown="Disabled" {
        disable-tunnel: [-2.25694 -3.5000000000000004 ("an 2")] -> w12
        frame Disabled {
        }
        frame Enabled {
        }
      }
      "an" <- w12
      n6 = global read "G_ALL.vi" "CARDATA"() -> (w5:T2)
      n7 = Unbundle By Name(w5) -> ("VS_can"=w17:dbl, "Steer_output"=w7:dbl)
      n8 = Divide(x=w7, y=w20) -> (x/y=w9:dbl)
      n9 = Divide(x=w17, y=3.6) -> (x/y=→"V":dbl)
      n10 = global read "G_ALL.vi" "CARSPEC"() -> (w4:T1)
      n11 = Multiply(x=w9, y=3.141592653589793) -> (x*y=w22:dbl)
      n12 = Unbundle By Name(w4) -> ("Overall width"=w1:dbl, "af"=→"af":dbl, "C_Wheel base"=w3:dbl)
      n13 = Divide(x=w22, y=180.0) -> (x/y=w8:dbl)
      n14 = Tangent(1:w8) -> (0:w11:dbl)
      n15 = Divide(x=w3, y=w11) -> (x/y=w14:dbl)
      n16 = Equal To 0?(x=w11) -> (x = 0?=→"straight":bool)
      n17 = Multiply(x=w1, y=0.5) -> (x*y=→"aw":dbl)
      n18 = Negate(x=w14) -> (-x=→"R":dbl)
      "ar" <- 0.75 ("af 2")
      "margin" <- 0.3 ("margin")
    }
    frame #1 {
      n19 = local read "margin"() -> (w54:dbl)
      n20 = local read "V"() -> (w44:dbl)
      n21 = local read "margin"() -> (w46:dbl)
      n22 = Greater Or Equal To 0?(x=w44) -> (x >= 0?=w30:bool)
      n23 = local read "R"() -> (w56:dbl)
      n24 = local read "aw"() -> (w53:dbl)
      n25 = local read "af"() -> (w43:dbl)
      n26 = local read "ar"() -> (w42:dbl)
      n27 = local read "aw"() -> (w47:dbl)
      n28 = local read "R"() -> (w45:dbl)
      n29 = local read "margin"() -> (w40:dbl)
      n30 = Select(t=w43, s=w30, f=w42) -> (s? t:f=w41:dbl)
      n31 = Add(x=w53, y=w54) -> (x+y=w52:dbl)
      n32 = Add(x=w47, y=w46) -> (x+y=w35:dbl)
      n33 = Absolute Value(x=w56) -> (abs(x)=w55:dbl)
      n34 = Absolute Value(x=w45) -> (abs(x)=w34:dbl)
      n35 = Sign(1:w56) -> (0:w50:dbl)
      n36 = Subtract(x=w55, y=w52) -> (x-y=w51:dbl)
      n37 = Add(x=w41, y=w40) -> (x+y=w31:dbl)
      n38 = Add(x=w35, y=w34) -> (x+y=w38:dbl)
      n39 = Square(x=w31) -> (x^2=w37:dbl)
      n40 = Square(x=w38) -> (x^2=w36:dbl)
      n41 = Multiply(x=w50, y=w51) -> (x*y=→"Rmin":dbl)
      n42 = Add(x=w37, y=w36) -> (x+y=w39:dbl)
      n43 = Square Root(x=w39) -> (sqrt(x)=w33:dbl)
      n44 = Sign(1:w45) -> (0:w32:dbl)
      n45 = Multiply(x=w33, y=w32) -> (x*y=→"Rmax":dbl)
    }
    frame #2 {
      n46 = disable-structure shown="Enabled" {
        disable-tunnel: [w58 w138] -> w57
        frame Enabled {
          n47 = flat-sequence {
            tunnel: [w62] -> w58
            frame #0 {
              n48 = disable-structure shown="Enabled" {
                disable-tunnel: [w68 _] -> w61
                frame Enabled {
                  n49 = global read "G_SEN.vi" "CIPV"() -> (w68:dbl[][])
                }
                frame Disabled {
                }
              }
              n50 = global read "G_SEN.vi" "sensor_obs"() -> (w65:dbl[][])
              n51 = Empty Array?(array=w61) -> (empty?=w60:bool)
              n52 = case shown="False" w60 {
                tunnel: w61 -> [w96 _]
                tunnel: w65 -> [w71 w98]
                tunnel: [w70 w98] -> w64
                tunnel: [w69 _] -> w59
                frame False {
                  n53 = Index Array(array=w96, index (row)=0) -> (element=w94:dbl[])  [unwired: 1 in]
                  n54 = Index Array(array=w94, index #1=3 ("index"), index #2=1 ("index"), index #3=2 ("index")) -> (element #1=w90:dbl, element #2=w75:dbl, element #3=w78:dbl)
                  n55 = Multiply(x=0.5, y=w90) -> (x*y=w82:dbl)
                  n56 = Multiply(x=10.0, y=w82) -> (x*y=w87:dbl)
                  n57 = Round Toward -Infinity(1:w87) -> (0:w86:dbl)
                  n58 = for {
                    N: w86 -> [_]
                    tunnel: [w97] -> w85 mode=indexing
                    i -> [w97]
                  }
                  n59 = Multiply(x=w85, y=0.1 ("x")) -> (x*y=w83:dbl[])
                  n60 = Build Array (concatenate)(w83, w82) -> (w79:dbl[])
                  n61 = Negate(x=w79) -> (-x=w81:dbl[])
                  n62 = Reverse 1D Array(array=w81) -> (reversed array=w80:dbl[])
                  n63 = Build Array (concatenate)(w80, w79) -> (w76:dbl[])
                  n64 = Add(x=w76, y=w75) -> (x+y=w74:dbl[])
                  n65 = Array Size(array=w76) -> (size(s)=w77:i32)
                  n66 = Initialize Array(w78, w77) -> (w73:dbl[])
                  n67 = Build Array(w74, w73) -> (w72:dbl[][])
                  n68 = Transpose 2D Array(2D array=w72) -> (transposed array=w69:dbl[][])
                  n69 = Build Array (concatenate)(w69, w71) -> (w70:dbl[][])
                }
                frame True {
                }
              }
              n70 = case shown="True" "obsclose" {
                tunnel: [_ w114] -> w66
                frame False {
                }
                frame True {
                  n71 = global read "G_ALL.vi" "CARDATA"() -> (w100:T2)
                  n72 = local read "margin"() -> (w103:dbl)
                  n73 = global read "G_SEN.vi" "sensor_obs_log"() -> (w125:dbl[][])
                  n74 = Unbundle By Name(w100) -> ("x"=w112:dbl, "y"=w113:dbl, "heading"=w128:dbl)
                  n75 = local read "aw"() -> (w104:dbl)
                  n76 = Add(x=w104, y=w103) -> (x+y=w102:dbl)
                  n77 = Negate(x=w128) -> (-x=w111:dbl)
                  n78 = local read "af"() -> (w99:dbl)
                  n79 = Index Array(array=w125, index (col) #1=0 ("disabled index (col)")) -> (element #1=w127:dbl[], element #2=w126:dbl[])  [unwired: 3 in]
                  n80 = Negate(x=w102) -> (-x=w101:dbl)
                  n81 = Add(x=3.0, y=w99) -> (x+y=w106:dbl)
                  n82 = call "rotm_mimo.vi"("angle[rad]"=w111, "reverse"=FALSE, "y0"=w113, "x0"=w112, "y"=w126, "x"=w127) -> ("Y"=w122:dbl[], "X"=w110:dbl[])  [unwired: 2 in, 2 out]
                  n83 = In Range and Coerce(upper limit=w106, x=w122, lower limit=w99) -> (In Range?=w108:bool[])  [unwired: 1 out]
                  n84 = In Range and Coerce(upper limit=w102, x=w110, lower limit=w101) -> (In Range?=w109:bool[])  [unwired: 1 out]
                  n85 = And(x=w108, y=w109) -> (x .and. y?=w107:bool[])
                  n86 = Boolean To (0,1)(Boolean=w107) -> (0, 1=w120:i16[])
                  n87 = Not(x=w107) -> (.not. x?=w124:bool[])
                  n88 = Add Array Elements(numeric array=w120) -> (sum=w119:i16)
                  n89 = Boolean To (0,1)(Boolean=w124) -> (0, 1=w123:i16[])
                  n90 = Build Cluster Array(w123, w110, w122) -> (w121:T3)
                  n91 = Sort 1D Array(array=w121) -> (sorted array=w118:T3)
                  n92 = for {
                    N: w119 -> [_]
                    tunnel: w118 -> [w133] mode=indexing
                    tunnel: [w132] -> w117 mode=indexing
                    tunnel: [w131] -> w116 mode=indexing
                    n93 = Unbundle(w133) -> ("Real Matrix Element"=w132:dbl, "Real Matrix Element"=w131:dbl)  [unwired: 1 out]
                  }
                  n94 = Build Array(w117, w116) -> (w115:dbl[][])
                  n95 = Transpose 2D Array(2D array=w115) -> (transposed array=w114:dbl[][])
                }
              }
              n96 = Empty Array?(array=w66) -> (empty?=w67:bool)
              n97 = case shown="True" w67 {
                tunnel: w66 -> [w136 _]
                tunnel: w64 -> [w135 w137]
                tunnel: [w134 w137] -> w62
                frame False {
                  n98 = Build Array (concatenate)(w136, w135) -> (w134:dbl[][])
                }
                frame True {
                }
              }
              n99 = global write "G_SEN.vi" "CIPV show"(w59) -> ()
            }
          }
        }
        frame Disabled {
          n100 = global read "G_SEN.vi" "sensor_obs"() -> (w138:dbl[][])
        }
      }
      "sensor" <- w57
    }
    frame #3 {
      n101 = local read "sensor"() -> (w140:dbl[][])
      n102 = Empty Array?(array=w140) -> (empty?=w139:bool)
      n103 = case shown="False" w139 {
        tunnel: [w145 _] -> w142
        tunnel: [w144 inf] -> w141
        frame False {
          n104 = local read "straight"() -> (w143:bool)
          n105 = case shown="False" w143 {
            tunnel: [w152 w231] -> w145
            tunnel: [w151 w230] -> w144
            frame False {
              n106 = local read "sensor"() -> (w176:dbl[][])
              n107 = Index Array(array=w176, index (col) #1=0 ("disabled index (col)"), index (col) #2=1 ("index (col)")) -> (element #1=w173:dbl[], element #2=w159:dbl[])  [unwired: 2 in]
              n108 = Square(x=w159) -> (x^2=w170:dbl[])
              n109 = local read "R"() -> (w172:dbl)
              n110 = Subtract(x=w173, y=w172) -> (x-y=w160:dbl[])
              n111 = local read "Rmax"() -> (w168:dbl)
              n112 = local read "Rmin"() -> (w169:dbl)
              n113 = Square(x=w160) -> (x^2=w171:dbl[])
              n114 = Square(x=w168) -> (x^2=w165:dbl)
              n115 = Square(x=w169) -> (x^2=w167:dbl)
              n116 = Add(x=w171, y=w170) -> (x+y=w166:dbl[])
              n117 = Greater Or Equal?(x=w165, y=w166) -> (x >= y?=w164:bool[])
              n118 = Greater Or Equal?(x=w166, y=w167) -> (x >= y?=w163:bool[])
              n119 = And(x=w164, y=w163) -> (x .and. y?=w162:bool[])
              n120 = Boolean To (0,1)(Boolean=w162) -> (0, 1=w161:i16[])
              n121 = Build Cluster Array(w161, w160, w159) -> (w158:cluster{i16, dbl, "element":dbl}[])
              n122 = Sort 1D Array(array=w158) -> (sorted array=w157:cluster{i16, dbl, "element":dbl}[])
              n123 = for {
                tunnel: w157 -> [w219] mode=indexing
                tunnel: [w218] -> w156 mode=indexing
                tunnel: [w217] -> w155 mode=indexing
                tunnel: [w216] -> w148 mode=indexing
                n124 = Unbundle(w219) -> (w218:i16, w217:dbl, "element"=w216:dbl)
              }
              n125 = Equal To 0?(x=w156) -> (x = 0?=w154:bool[])
              n126 = Boolean To (0,1)(Boolean=w154) -> (0, 1=w153:i16[])
              n127 = Add Array Elements(numeric array=w153) -> (sum=w147:i16)
              n128 = Array Subset(array=w155, index=w147) -> (w150:dbl[])  [unwired: 1 in]
              n129 = Array Subset(array=w148, index=w147) -> (w146:dbl[])  [unwired: 1 in]
              n130 = Empty Array?(array=w150) -> (empty?=w149:bool)
              n131 = case shown="False" w149 {
                tunnel: w150 -> [w192 _]
                tunnel: [w184 _] -> w152
                tunnel: [w182 inf] -> w151
                tunnel: w146 -> [w178 _]
                frame False {
                  n132 = local read "R"() -> (w196:dbl)
                  n133 = local read "R"() -> (w180:dbl)
                  n134 = Add(x=w192, y=w196) -> (x+y=w195:dbl[])
                  n135 = Sign(1:w180) -> (0:w181:dbl)
                  n136 = Negate(x=w181) -> (-x=w179:dbl)
                  n137 = Build Array(w195, w178) -> (w194:dbl[][])
                  n138 = Multiply(x=w192, y=w179) -> (x*y=w191:dbl[])
                  n139 = local read "V"() -> (w190:dbl)
                  n140 = Re/Im To Polar(2:w178, 3:w191) -> (0:w193:dbl[], 1:w189:dbl[])
                  n141 = Greater Or Equal To 0?(x=w190) -> (x >= 0?=w177:bool)
                  n142 = Transpose 2D Array(2D array=w194) -> (transposed array=w186:dbl[][])
                  n143 = case shown="True" w177 {
                    tunnel: w193 -> [w200 w209]
                    tunnel: [w198 w207] -> w187
                    tunnel: [w197 w206] -> w185
                    frame True {
                      n144 = for {
                        tunnel: w200 -> [w205] mode=indexing
                        tunnel: [w204] -> w199 mode=indexing
                        n145 = Less Than 0?(x=w205) -> (x < 0?=w203:bool)
                        n146 = Add(x=6.283185307179586, y=w205) -> (x+y=w201:dbl)
                        n147 = Select(t=w201, s=w203, f=w205) -> (s? t:f=w204:dbl)
                      }
                      n148 = Array Max & Min(array=w199) -> (min value=w198:dbl, min index (indices)=w197:i32)  [unwired: 2 out]
                    }
                    frame False {
                      n149 = for {
                        tunnel: w209 -> [w214] mode=indexing
                        tunnel: [w213] -> w208 mode=indexing
                        n150 = Less Than 0?(x=w214) -> (x < 0?=w212:bool)
                        n151 = Subtract(x=w214, y=6.283185307179586) -> (x-y=w210:dbl)
                        n152 = Select(t=w214, s=w212, f=w210) -> (s? t:f=w213:dbl)
                      }
                      n153 = Array Max & Min(array=w208) -> (max value=w207:dbl, max index (indices)=w206:i32)  [unwired: 2 out]
                    }
                  }
                  n154 = Index Array(array=w186, index (row)=w185) -> (element=w184:dbl[])  [unwired: 1 in]
                  n155 = Index Array(array=w189, index=w185) -> (element=w188:dbl)
                  n156 = Multiply(x=w188, y=w187) -> (x*y=w183:dbl)
                  n157 = Absolute Value(x=w183) -> (abs(x)=w182:dbl)
                }
                frame True {
                }
              }
            }
            frame True {
              n158 = local read "margin"() -> (w225:dbl)
              n159 = local read "aw"() -> (w226:dbl)
              n160 = local read "sensor"() -> (w245:dbl[][])
              n161 = Add(x=w226, y=w225) -> (x+y=w224:dbl)
              n162 = Negate(x=w224) -> (-x=w223:dbl)
              n163 = Index Array(array=w245, index (col) #1=0 ("disabled index (col)"), index (col) #2=1 ("index (col)")) -> (element #1=w227:dbl[], element #2=w238:dbl[])  [unwired: 2 in]
              n164 = Greater Or Equal?(x=w224, y=w227) -> (x >= y?=w242:bool[])
              n165 = Greater Or Equal?(x=w227, y=w223) -> (x >= y?=w241:bool[])
              n166 = And(x=w242, y=w241) -> (x .and. y?=w240:bool[])
              n167 = Boolean To (0,1)(Boolean=w240) -> (0, 1=w239:i16[])
              n168 = Build Cluster Array(w239, w227, w238) -> (w237:cluster{i16, "element":dbl, "element":dbl}[])
              n169 = Sort 1D Array(array=w237) -> (sorted array=w236:cluster{i16, "element":dbl, "element":dbl}[])
              n170 = for {
                tunnel: w236 -> [w276] mode=indexing
                tunnel: [w275] -> w235 mode=indexing
                tunnel: [w274] -> w234 mode=indexing
                tunnel: [w273] -> w222 mode=indexing
                n171 = Unbundle(w276) -> (w275:i16, "element"=w274:dbl, "element"=w273:dbl)
              }
              n172 = Equal To 0?(x=w235) -> (x = 0?=w233:bool[])
              n173 = Boolean To (0,1)(Boolean=w233) -> (0, 1=w232:i16[])
              n174 = Add Array Elements(numeric array=w232) -> (sum=w221:i16)
              n175 = Array Subset(array=w234, index=w221) -> (w229:dbl[])  [unwired: 1 in]
              n176 = Array Subset(array=w222, index=w221) -> (w220:dbl[])  [unwired: 1 in]
              n177 = Empty Array?(array=w229) -> (empty?=w228:bool)
              n178 = case shown="False" w228 {
                tunnel: w229 -> [w249 _]
                tunnel: [w251 _] -> w231
                tunnel: [w250 inf] -> w230
                tunnel: w220 -> [w248 _]
                frame False {
                  n179 = Build Array(w249, w248) -> (w255:dbl[][])
                  n180 = local read "V"() -> (w254:dbl)
                  n181 = Greater Or Equal To 0?(x=w254) -> (x >= 0?=w246:bool)
                  n182 = case shown="True" w246 {
                    tunnel: [w258 w266] -> w252
                    tunnel: w248 -> [w257 w265]
                    tunnel: [w256 w264] -> w247
                    frame True {
                      n183 = for {
                        tunnel: w257 -> [w263] mode=indexing
                        tunnel: [w262] -> w259 mode=indexing
                        n184 = Greater Or Equal To 0?(x=w263) -> (x >= 0?=w261:bool)
                        n185 = Select(t=w263, s=w261, f=inf) -> (s? t:f=w262:dbl)
                      }
                      n186 = Array Max & Min(array=w259) -> (min value=w256:dbl, min index (indices)=w258:i32)  [unwired: 2 out]
                    }
                    frame False {
                      n187 = for {
                        tunnel: w265 -> [w271] mode=indexing
                        tunnel: [w270] -> w267 mode=indexing
                        n188 = Less Than 0?(x=w271) -> (x < 0?=w269:bool)
                        n189 = Select(t=w271, s=w269, f=-inf) -> (s? t:f=w270:dbl)
                      }
                      n190 = Array Max & Min(array=w267) -> (max value=w264:dbl, max index (indices)=w266:i32)  [unwired: 2 out]
                    }
                  }
                  n191 = Transpose 2D Array(2D array=w255) -> (transposed array=w253:dbl[][])
                  n192 = Absolute Value(x=w247) -> (abs(x)=w250:dbl)
                  n193 = Index Array(array=w253, index (row)=w252) -> (element=w251:dbl[])  [unwired: 1 in]
                }
                frame True {
                }
              }
            }
          }
        }
        frame True {
        }
      }
      "coldist" <- w141
      "col point" <- w142
    }
    frame #4 {
      n194 = local read "sensor"() -> (w305:dbl[][])
      n195 = local read "coldist"() -> (w300:dbl)
      "collision dist" <- w300
      n196 = Empty Array?(array=w305) -> (empty?=w304:bool)
      n197 = feedback #1(w300) -> (w298:dbl)
      n198 = feedback-in #1(w300) -> ()
      n199 = Less?(x=w300, y=w298) -> (x < y?=w301:bool)
      n200 = case shown="False" w304 {
        tunnel: [w314 _] -> w279
        frame False {
          n201 = local read "col point"() -> (w317:dbl[])
          n202 = Empty Array?(array=w317) -> (empty?=w316:bool)
          n203 = Index Array(array=w317, index #1=0 ("index")) -> (element #1=w319:dbl, element #2=w318:dbl)  [unwired: 1 in]
          n204 = global read "G_ALL.vi" "xobs"() -> (w313:cluster{"idx":i32, "x":dbl, "y":dbl, "h":dbl})
          n205 = Bundle By Name(cluster=w313, "idx"=1 ("c_idx"), "x"=w319, "y"=w318) -> (w315:cluster{"idx":i32, "x":dbl, "y":dbl, "h":dbl})
          n206 = Select(t=cluster{"idx":i32, "x":dbl, "y":dbl, "h":dbl} {"idx"=0, "x"=0.0, "y"=0.0, "h"=0.0} ("xobs"), s=w316, f=w315) -> (s? t:f=w314:cluster{"idx":i32, "x":dbl, "y":dbl, "h":dbl})
        }
        frame True {
        }
      }
      n207 = feedback #2(w298) -> (w297:dbl)
      n208 = feedback-in #2(w298) -> ()
      n209 = Less?(x=w298, y=w297) -> (x < y?=w299:bool)
      n210 = Select(t=w298, s=w299, f=w297) -> (s? t:f=w296:dbl)
      n211 = Select(t=w300, s=w301, f=w296) -> (s? t:f=w291:dbl)
      n212 = Max & Min(x=w291, y=200.0) -> (min(x,y)=w287:dbl)  [unwired: 1 out]
      n213 = local read "V"() -> (w289:dbl)
      n214 = Multiply(x="y", y=w289) -> (x*y=w284:dbl)
      n215 = Multiply(x=w287, y="y") -> (x*y=w285:dbl)
      n216 = Max & Min(x=w285, y=w284) -> (max(x,y)=w286:dbl)  [unwired: 1 out]
      n217 = global write "G_ALL.vi" "xobs"(w279) -> ()
      n218 = local read "af"() -> (w278:dbl)
      n219 = Compound Arithmetic op=ADD(w286, "safe  dist", w278) -> (w292:dbl)
      n220 = Subtract(x=w291, y=w292) -> (x-y=w283:dbl)
      n221 = Multiply(x=w283, y=20.0) -> (x*y=w281:dbl)
      n222 = Square Root(x=w281) -> (sqrt(x)=w280:dbl)
      n223 = Max & Min(x=w280, y=0.0) -> (max(x,y)=w307:dbl)  [unwired: 1 out]
      n224 = local read "V"() -> (w290:dbl)
      n225 = Multiply(x=w307, y=3.6) -> (x*y=w303:dbl)
      n226 = Greater?(x=w290, y=w307) -> (0:→"collision":bool)
      n227 = Build Array("Max. Vel.", w303) -> (w309:dbl[])
      n228 = Absolute Value(x=w309) -> (abs(x)=w310:dbl[])
      n229 = Array Max & Min(array=w310) -> (min value=→"speed limit":dbl)  [unwired: 3 out]
    }
  }
